vi "DI.vi"(11 "DAQ数字采集通道参数设置":T1={"数据采集设置"={"lines"="", "line grouping"=1}, "采样设置"={"rate"=1000.0, "sample mode"=10178, "samples per channel"=1000}, "ConvLateErrorsToWarnings"=FALSE} {"采样设置"."sample mode" items=["Finite Samples"=10178, "Continuous Samples"=10123, "Hardware Timed Single Point"=12522]; "采样设置"."rate" format="%0.2f"; "数据采集设置"."line grouping" items=["one channel for each line", "one channel for all lines"]}) -> (0 "error out":errorcluster, 3 "task out":refnum<k21>)   [LabVIEW 2018]
uses:
  <vilib>/DAQmx/create/channels.llb/DAQmx Create Channel (DI-Digital Input).vi
  <vilib>/DAQmx/configure/timing.llb/DAQmx Timing (Sample Clock).vi
  <resource>/objmgr/daqmx.rc
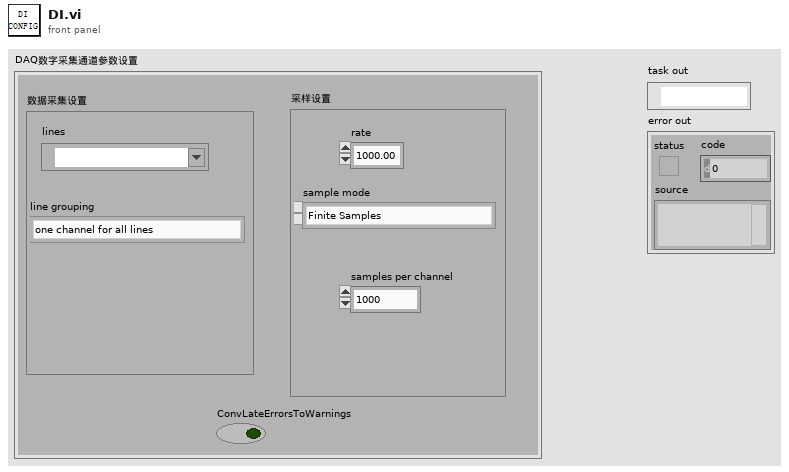
[diagram p1: front panel]
types:
  T1 = cluster{"数据采集设置":cluster{"lines":tag, "line grouping":i32}, "采样设置":cluster{"rate":dbl, "sample mode":i32, "samples per channel":i32}, "ConvLateErrorsToWarnings":bool}
  T2 = cluster{"rate":dbl, "sample mode":i32, "samples per channel":i32}
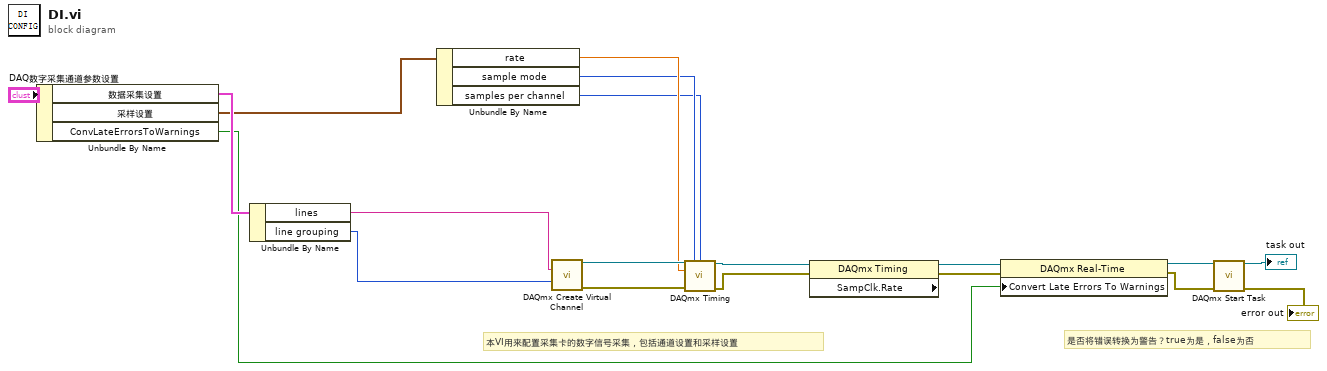
[diagram p0: block diagram]
diagram:
  # "是否将错误转换为警告？true为是，false为否"
  # "本VI用来配置采集卡的数字信号采集，包括通道设置和采样设置"
  n1 = Unbundle By Name("DAQ数字采集通道参数设置") -> ("数据采集设置"=w3:cluster{"lines":tag, "line grouping":i32}, "采样设置"=w2:T2, "ConvLateErrorsToWarnings"=w1:bool)
  n2 = Unbundle By Name(w3) -> ("lines"=w6:tag, "line grouping"=w5:i32)
  n3 = Unbundle By Name(w2) -> ("rate"=w9:dbl, "sample mode"=w8:i32, "samples per channel"=w7:i32)
  n4 = call-poly <vilib>:"DAQmx Create Virtual Channel.vi"("lines"=w6, "line grouping"=w5) -> ("task out"=w17:refnum<k21>, "error out"=w16:errorcluster)  [unwired: 12 in]
  n5 = call-poly <vilib>:"DAQmx Timing.vi"("task/channels in"=w17, "sample mode"=w8, "samples per channel"=w7, "rate"=w9, "error in"=w16) -> ("task out"=w15:refnum<k21>, "error out"=w14:errorcluster)  [unwired: 9 in]
  n6 = property class="DAQmx Timing" props=["SampClk.Rate"](reference=w15, error in=w14) -> (reference out=w19:refnum<k21>, error out=w18:errorcluster)  [unwired: 1 out]
  n7 = property class="DAQmx Real-Time"(reference=w19, error in=w18, "Convert Late Errors To Warnings"=w1) -> (reference out=w13:refnum<k21>, error out=w12:errorcluster)
  n8 = call <vilib>:"DAQmx Start Task.vi"("task/channels in"=w13, "error in"=w12) -> ("task out"=→"task out":refnum<k21>, "error out"=→"error out":errorcluster)  [unwired: 12 in]
